vi "ClassesOverview.vi"() -> (0 "error out":errorcluster)   [LabVIEW 2016]
uses:
  <resource>/Framework/Providers/Open_GDS/ClassProviders/Common/LvClass_class/GDSLvCLass_ClassSettingsType.ctl
  <resource>/Framework/Providers/Open_GDS/ClassProviders/Common/LvClass_class/GDSLvClass_PlugIn.ctl
  <resource>/Framework/Providers/Open_GDS/ClassProviders/Common/LvClass_class/GDSLvClass_PlugInTypes.ctl
  <resource>/Framework/Providers/Open_GDS/ClassProviders/Provider_BaseClassInterface/ClassWriter_class/ClassWriter.lvclass
  <vilib>/Utility/miscctls.llb/LVPositionTypeDef.ctl
  <vilib>/Utility/error.llb/DialogType.ctl
panel:
  in  "OnlyClassesThatNeedsToBeUpdated":bool=TRUE
  out "Slide":u8(slide) scale=0.0..100.0
  in  "Done":bool
  in  "UpdateSelected":bool
  in  "Classes":i32[](listbox)
  in  "Cancel":bool
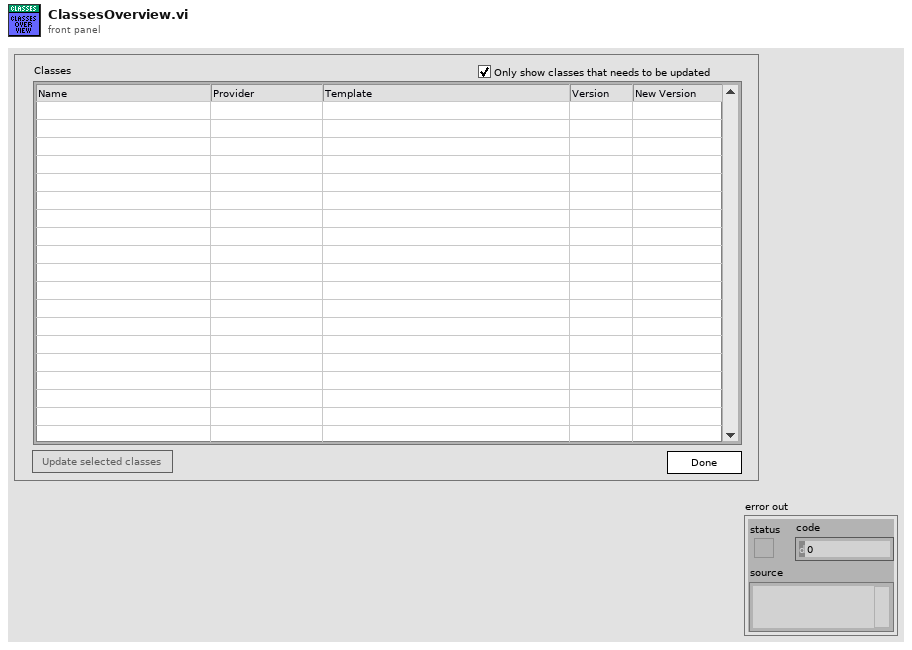
[diagram p1: front panel]
types:
  T1 = typedef "GDSLvCLass_ClassSettingsType.ctl" = cluster{"ClassProviderName":string, "ClassTemplateUsed":string, "ClassTemplateVersion":string, "ClassDescription":string, "PlugIns":T2[], "ConnectorPanePattern":string}
  T2 = typedef "GDSLvClass_PlugIn.ctl" = cluster{"Type":T3, "ID":string, "Version":string, "Path":path, "Name":string, "Data":variant}
  T3 = typedef "GDSLvClass_PlugInTypes.ctl" = enum16{"DesignPattern", "MethodTypes"}
  T4 = cluster{"ClassInfo":T1[], "Classes":refnum<vi>[], "NewVersions":string[], "ClassWriters":refnum<class "ClassWriter.lvclass">[]}
  T5 = typedef "LVPositionTypeDef.ctl" = cluster{"Left":i32, "Top":i32}
  T6 = cluster{"Major":u16, "Minor":u16, "Fix":u16, "Build":u16}
  T7 = typedef "DialogType.ctl" = u16
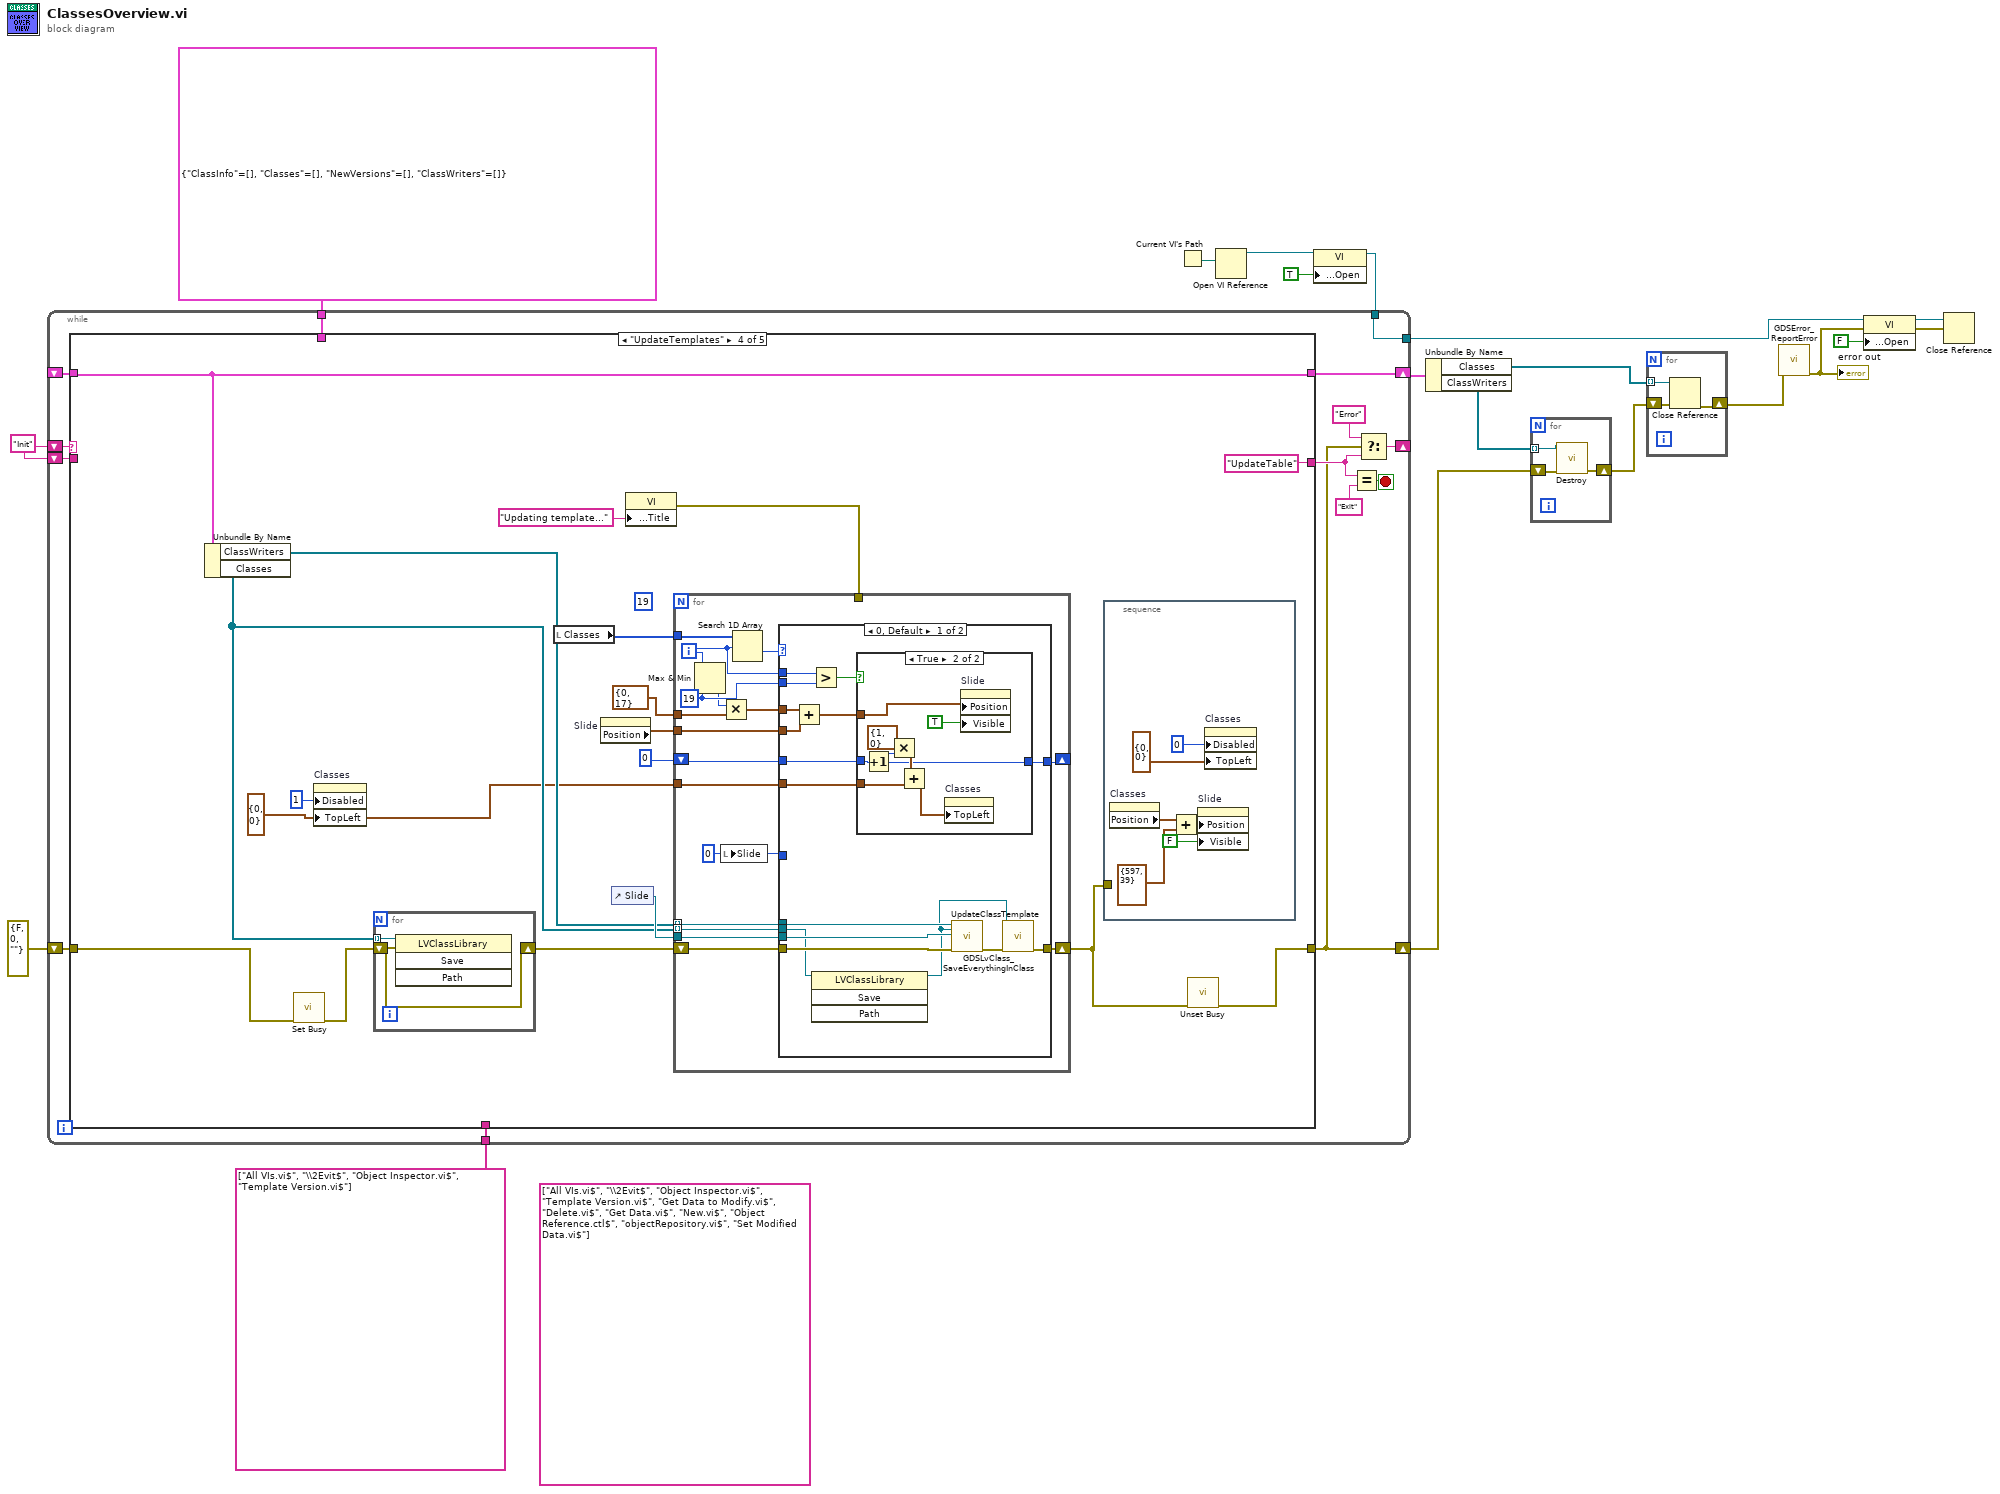
[diagram p0: block diagram]
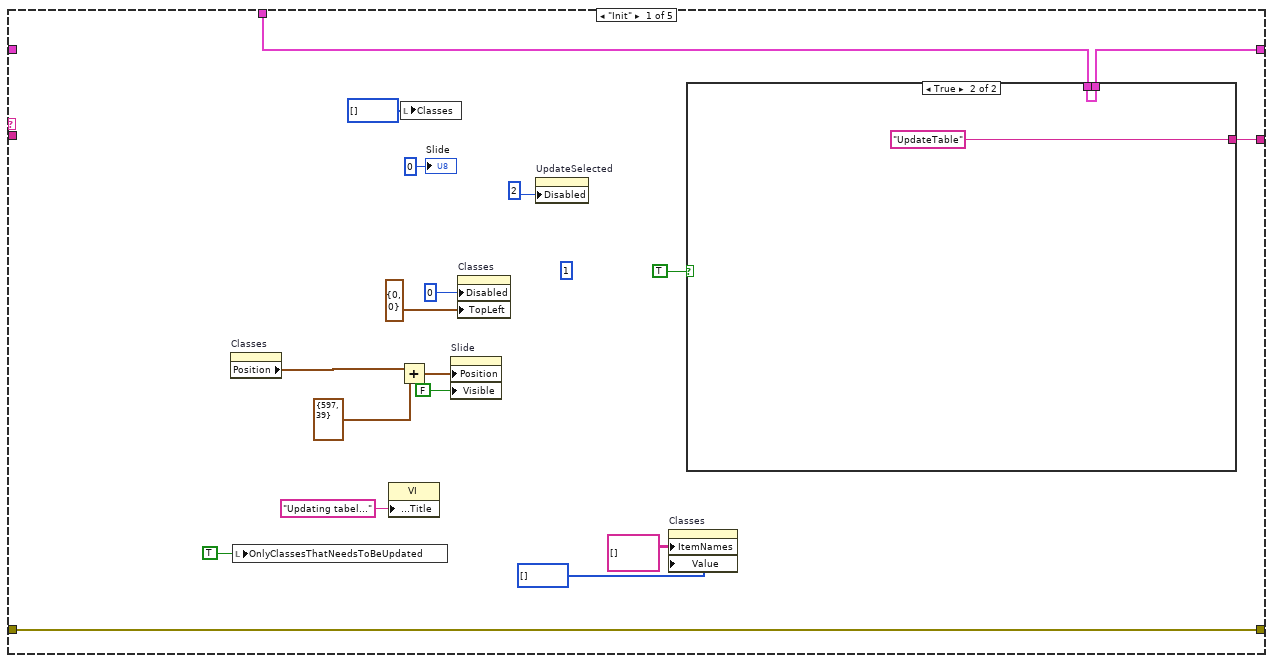
[diagram p2: hidden frame]
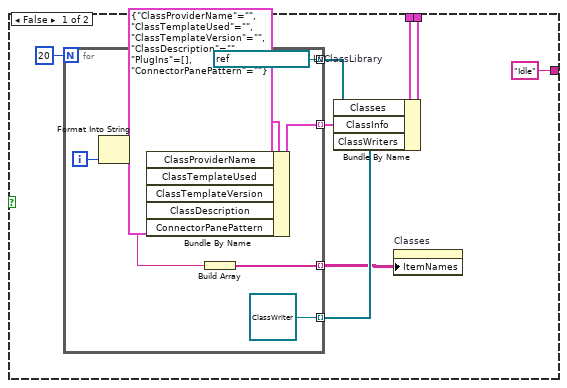
[diagram p3: hidden frame]
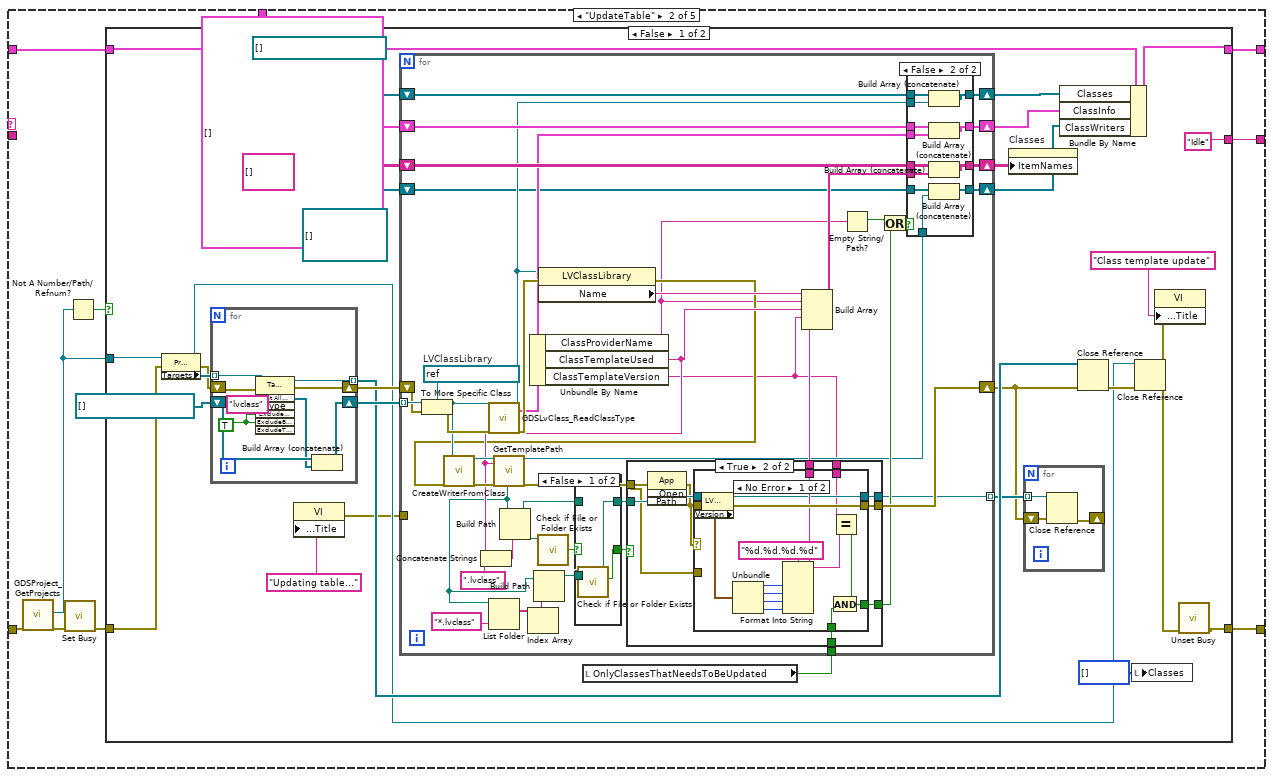
[diagram p4: hidden frame]
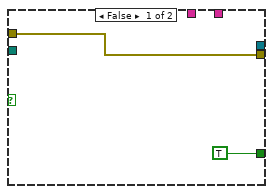
[diagram p6: hidden frame]
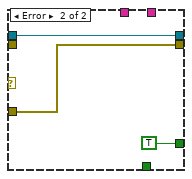
[diagram p7: hidden frame]
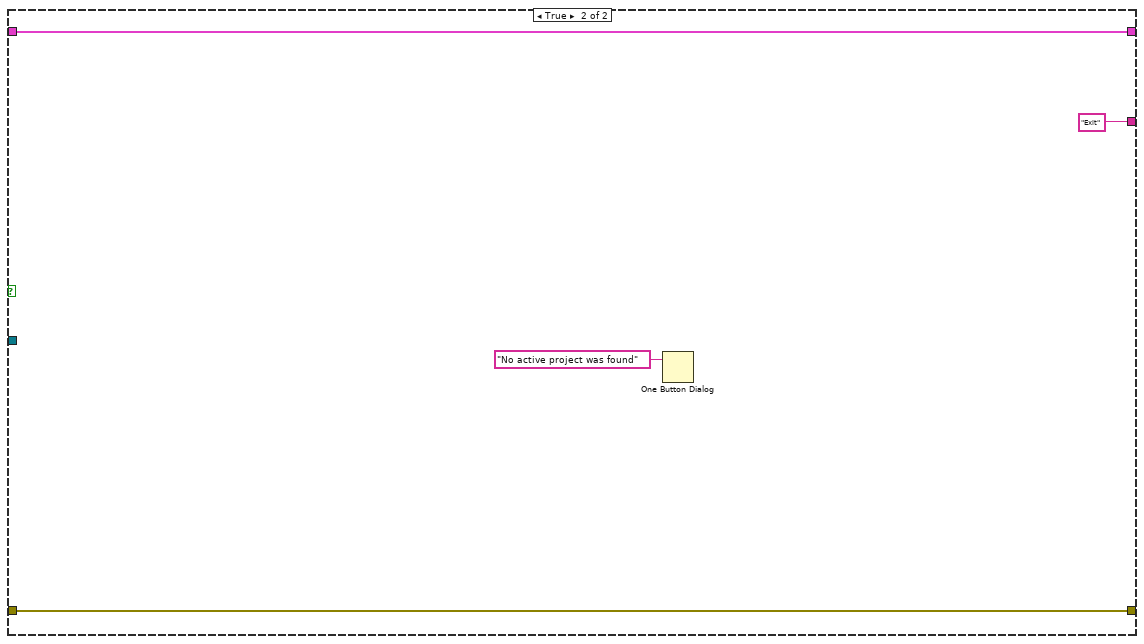
[diagram p9: hidden frame]
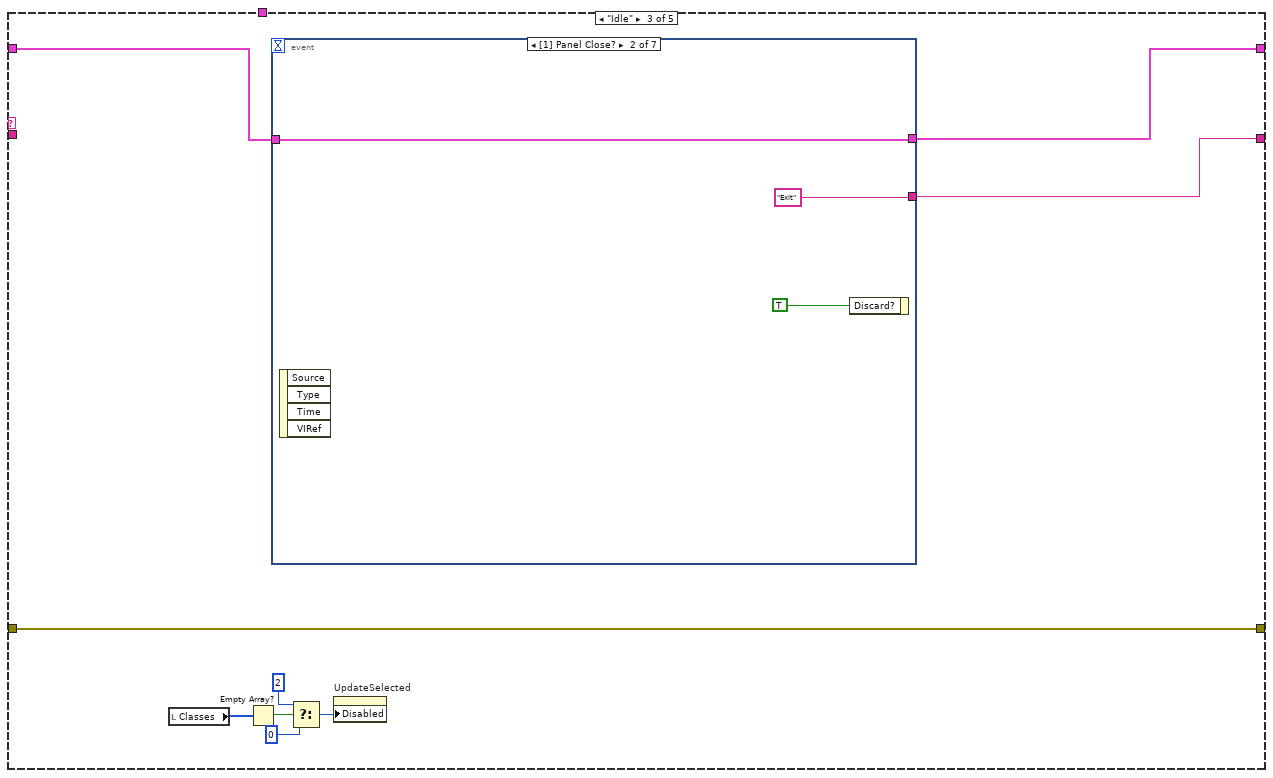
[diagram p10: hidden frame]
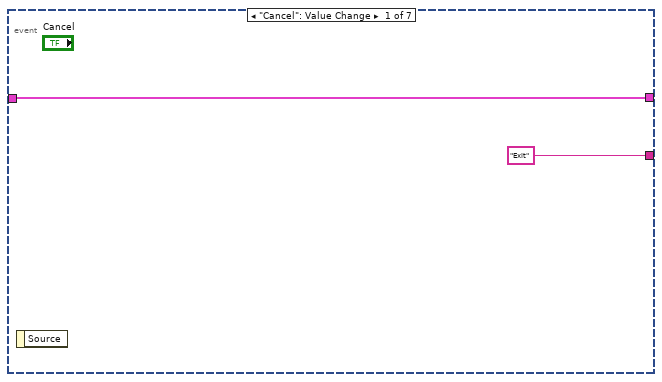
[diagram p11: hidden frame]
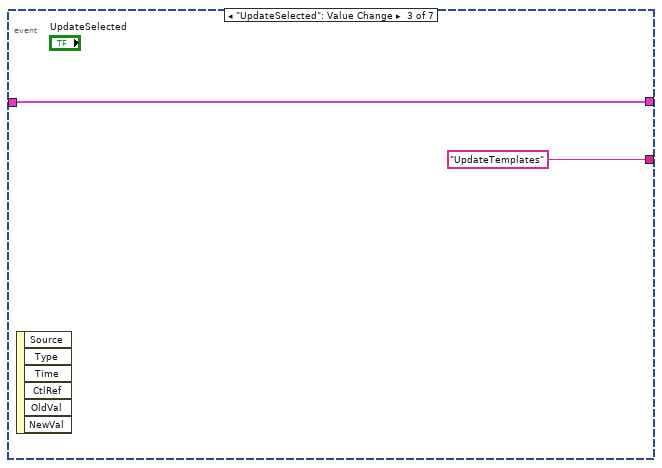
[diagram p12: hidden frame]
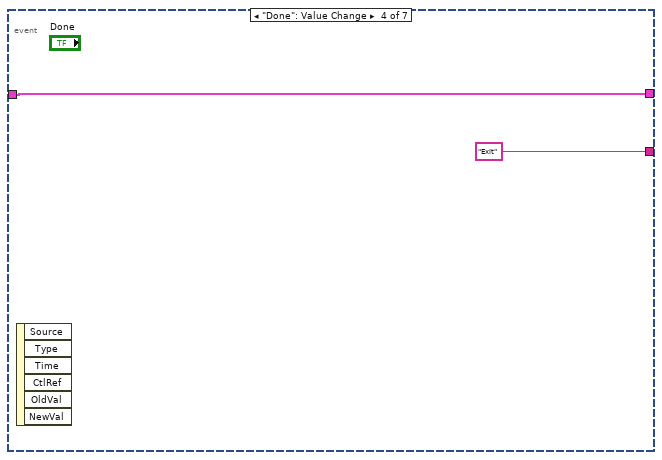
[diagram p13: hidden frame]
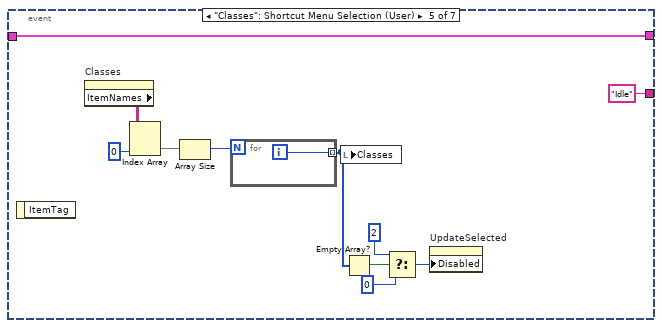
[diagram p14: hidden frame]
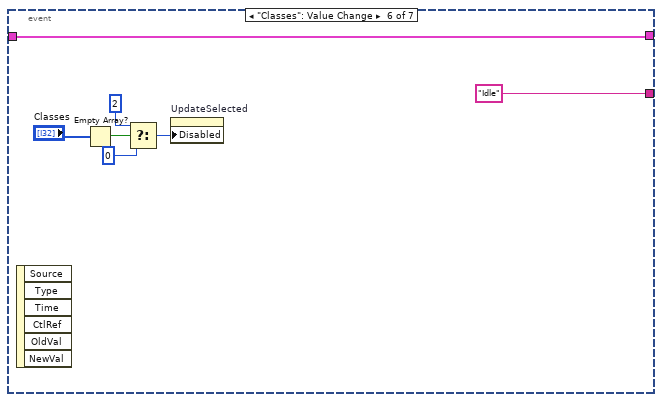
[diagram p15: hidden frame]
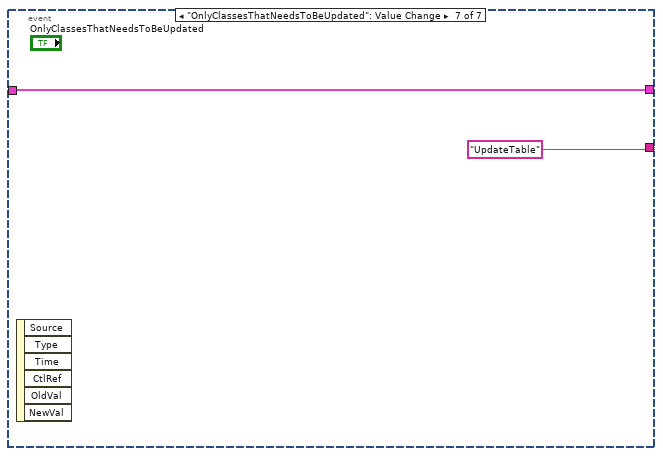
[diagram p16: hidden frame]
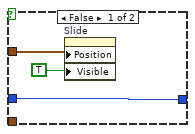
[diagram p17: hidden frame]
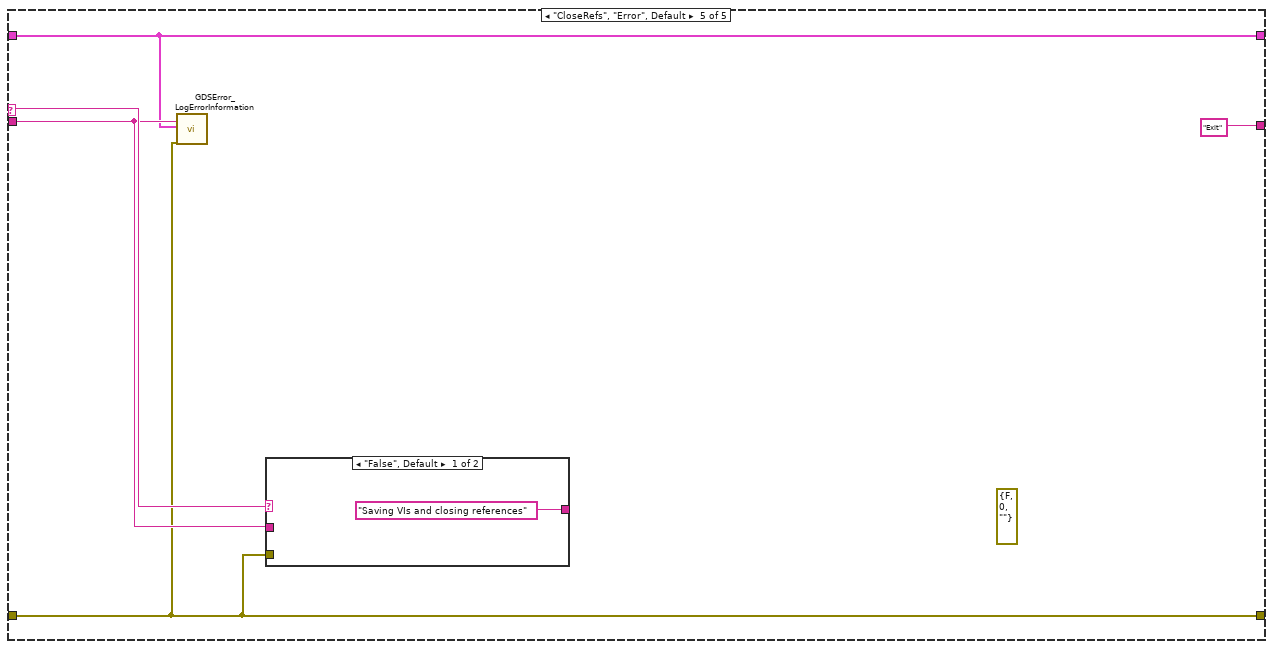
[diagram p19: hidden frame]
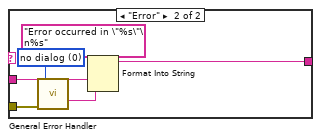
[diagram p20: hidden frame]
diagram:
  (unwired) string[] ["All VIs.vi$", "\\2Evit$", "Object Inspector.vi$", "Template Version.vi$", "Get Data to Modify.vi$", "Delete.vi$", "Get Data.vi$", "New.vi$", "Object Reference.ctl$", "objectRepository.vi$", "Set Modified Data.vi$"] ("file names")
  w17 = "Init"
  n1 = Current VI's Path() -> (path=w16:path)
  n2 = Open VI Reference(vi path=w16) -> (vi reference=w15:refnum<vi>)  [unwired: 5 in, 1 out]
  n3 = property class="VI"(reference=w15, "Front Panel.Open"=TRUE ("Front Panel Window:Open")) -> (reference out=w14:refnum<vi>)  [unwired: 1 in, 1 out]
  n4 = while {
    shift-right: [w27] -> w3
    shift-left: errorcluster {"status"=FALSE, "code"=0, "source"=""} ("error IO") -> [w33]
    shift-right: [w32] -> _
    shift-left: w17 -> [w21]
    shift-right: [w26] -> w6
    shift-left: _ -> [w25]
    tunnel: T4 {"ClassInfo"=[], "Classes"=[], "NewVersions"=[], "ClassWriters"=[]} -> [w24]
    tunnel: string[] ["All VIs.vi$", "\\2Evit$", "Object Inspector.vi$", "Template Version.vi$"] ("file names") -> [w23]
    shift-left: w17 -> [w22]
    tunnel: w14 -> [w20]
    tunnel: [w20] -> w9
    stop <- w31 stop-if-true
    n5 = case shown="\"UpdateTemplates\"" w21 {
      selector: w21 -> [_ _ _ _ w333]
      tunnel: w33 -> [w51 w77 w224 w263 w330]
      tunnel: [w51 w74 w224 w265 w330] -> w27
      tunnel: [w47 w75 w225 "UpdateTable" "Exit"] -> w28
      tunnel: [w38 w73 w226 w275 w331] -> w26
      tunnel: w25 -> [_ w72 w227 w275 w331]
      tunnel: w24 -> [w39 _ _ _ _]
      tunnel: w23 -> [_ _ _ _ _]
      tunnel: w22 -> [_ _ _ _ w332]
      frame "Init" {
        (unwired) u8 1 ("Disabled")
        n6 = property on="Classes" class="MCListbox (strict)"() -> ("Position"=w42:T5)  [unwired: 2 in, 2 out]
        n7 = local write "OnlyClassesThatNeedsToBeUpdated"(TRUE ("OnlyClassesThatNeedsToBeUpdated")) -> ()
        n8 = property class="VI"("Front Panel.Title"="Updating tabel..." ("Front Panel Window:Title")) -> ()  [unwired: 2 in, 2 out]
        n9 = Add(x=w42, y=T5 {"Left"=597, "Top"=39} ("x-y")) -> (x+y=w50:T5)
        n10 = local write "Classes"(i32[] [] ("Classes")) -> ()
        n11 = property on="Slide" class="Slide (strict)"("Position"=w50, "Visible"=FALSE) -> ()  [unwired: 2 in, 2 out]
        n12 = property on="Classes" class="MCListbox (strict)"("Disabled"=u8 0, "TopLeft"=cluster{"Row":u32, "Column":u32} {"Row"=0, "Column"=0} ("Top Left Visible Cell")) -> ()  [unwired: 2 in, 2 out]
        n13 = property on="UpdateSelected" class="Bool"("Disabled"=u8 2) -> ()  [unwired: 2 in, 2 out]
        n14 = property on="Classes" class="MCListbox (strict)"("ItemNames"=string[][] [] ("Item Names"), "Value"=i32[] [] ("Classes")) -> ()  [unwired: 2 in, 2 out]
        n15 = case shown="True" TRUE {
          tunnel: ["Idle" "UpdateTable"] -> w47
          tunnel: w39 -> [w58 w67]
          tunnel: [w57 w67] -> w38
          frame False {
            n16 = for {
              N: 20 -> [_]
              tunnel: [w66] -> w55 mode=indexing
              tunnel: [refnum<class "ClassWriter.lvclass"> refnum ("ClassWriterOut")] -> w54 mode=indexing
              tunnel: [w63] -> w53 mode=indexing
              tunnel: [w60] -> w52 mode=indexing
              i -> [w62]
              w66 = refnum<vi> refnum  # LVClassLibrary
              n17 = Format Into String(w62) -> (resulting string=w61:string)  [unwired: 3 in, 1 out]
              n18 = Bundle By Name(cluster=T1 {"ClassProviderName"="", "ClassTemplateUsed"="", "ClassTemplateVersion"="", "ClassDescription"="", "PlugIns"=[], "ConnectorPanePattern"=""} ("input cluster"), "ClassProviderName"=w61, "ClassTemplateUsed"=w61, "ClassTemplateVersion"=w61, "ClassDescription"=w61, "ConnectorPanePattern"=w61) -> (w63:T1)
              n19 = Build Array(w61) -> (w60:string[])
            }
            n20 = Bundle By Name(cluster=w58, "Classes"=w55, "ClassInfo"=w53, "ClassWriters"=w54) -> (w57:T4)
            n21 = property on="Classes" class="MCListbox (strict)"("ItemNames"=w52) -> ()  [unwired: 2 in, 2 out]
          }
          frame True {
          }
        }
        "Slide" <- u8 0 ("Slide")
      }
      frame "UpdateTable" {
        n22 = call <resource>:"GDSProject_GetProjects.vi"("error in (no error)"=w77) -> ("Project Refnum"=w71:refnum<vi>, "error out"=w70:errorcluster)  [unwired: 16 in, 1 out]
        n23 = call <vilib>:"Set Busy.vi"("error in (no error)"=w70) -> ("error out"=w69:errorcluster)  [unwired: 9 in, 1 out]
        n24 = Not A Number/Path/Refnum?(number/path/refnum=w71) -> (NaN/Path/Refnum?=w76:bool)
        n25 = case shown="False" w76 {
          tunnel: w69 -> [w106 w217]
          tunnel: ["Idle" "Exit"] -> w75
          tunnel: [w80 w217] -> w74
          tunnel: [w98 w215] -> w73
          tunnel: w72 -> [w102 w215]
          tunnel: w71 -> [w107 _]
          frame False {
            n26 = property class="Project"(reference=w107, error in=w106) -> (reference out=w99:refnum<vi>, error out=w78:errorcluster, "Targets"=w105:refnum<vi>[])
            n27 = for {
              tunnel: w105 -> [w116] mode=indexing
              tunnel: [w111] -> w101 mode=indexing
              shift-right: [w108] -> w104
              shift-left: refnum<vi>[] [] -> [w110]
              shift-right: [w112] -> w103
              shift-left: w78 -> [w114]
              w113 = TRUE ("ExcludeDependencies")
              n28 = invoke class="TargetItem" method="Get All Descendents"(reference=w116, error in=w114, "Type"="lvclass", "Exclude Dependencies"=w113, "ExcludeBuilds"=w113) -> (reference out=w111:refnum<vi>, error out=w112:errorcluster, "All Descendents"=w109:refnum<vi>[])  [unwired: 2 in, 4 out]
              n29 = Build Array (concatenate)(w110, w109) -> (w108:refnum<vi>[])
            }
            n30 = property class="VI"("Front Panel.Title"="Updating table..." ("Front Panel Window:Title")) -> (error out=w82:errorcluster)  [unwired: 2 in, 1 out]
            n31 = local read "OnlyClassesThatNeedsToBeUpdated"() -> (w86:bool)
            n32 = for {
              tunnel: w104 -> [w163] mode=indexing
              shift-right: [w140] -> w91
              shift-left: w103 -> [w161]
              shift-right: [w156] -> w97
              shift-left: string[][] [] -> [w157]
              shift-right: [w154] -> w89
              shift-left: T1[] [] ("ClassInfo") -> [w153]
              shift-right: [w151] -> w93
              shift-left: refnum<vi>[] [] ("Classes") -> [w152]
              tunnel: [w134] -> w92 mode=indexing
              shift-right: [w132] -> w87
              shift-left: refnum<class "ClassWriter.lvclass">[] [] ("ClassWriters") -> [w133]
              tunnel: w86 -> [w129]
              tunnel: w82 -> [_]
              w162 = refnum<vi> refnum  # LVClassLibrary
              n33 = To More Specific Class(target class=w162, reference=w163, error in=w161) -> (specific class reference=w143:refnum<vi>, error out=w160:errorcluster)
              n34 = call <resource>:"GDSLvClass_ReadClassType.vi"("Class Refnum In"=w143, "error in (no error)"=w160) -> ("Class Refnum Out"=w149:refnum<vi>, "ClassSettings"=w150:T1, "error out"=w158:errorcluster)  [unwired: 15 in]
              n35 = Unbundle By Name(w150) -> ("ClassProviderName"=w138:string, "ClassTemplateUsed"=w142:string, "ClassTemplateVersion"=w130:string)
              n36 = Concatenate Strings(w142, ".lvclass" ("string")) -> (w148:string)
              n37 = property class="LVClassLibrary"(reference=w149, error in=w158) -> (error out=w141:errorcluster, "Name"=w159:string)  [unwired: 1 out]
              n38 = call <resource>:"CreateWriterFromClass.vi"("ClassPath/LvClassRef"=w143, "error in"=w141) -> ("ClassWriter"=w145:refnum<class "ClassWriter.lvclass">, "error out"=w144:errorcluster)  [unwired: 15 in, 1 out]
              n39 = call-dynamic "GetTemplatePath.vi"("ClassWriterIn"=w145, "ClassTemplateSubDirectory"=w142, "error in (no error)"=w144) -> ("ClassWriterOut"=w131:refnum<class "ClassWriter.lvclass">, "FolderPathOut"=w121:path, "error out"=w146:errorcluster)  [unwired: 12 in, 2 out]
              n40 = List Folder(path=w121, pattern="*.lvclass" ("string")) -> (filenames=w123:string[])  [unwired: 2 in, 3 out]
              n41 = Build Path(base path=w121, name or relative path=w148) -> (appended path=w126:path)
              n42 = Index Array(array=w123) -> (element=w122:string)  [unwired: 1 in]
              n43 = Build Path(base path=w121, name or relative path=w122) -> (appended path=w120:path)
              n44 = call <vilib>:"Check if File or Folder Exists.vi"("path"=w126) -> ("file or folder exists?"=w127:bool)  [unwired: 8 in, 2 out]
              n45 = case shown="False" w127 {
                selector: w127 -> [_ w168]
                tunnel: w126 -> [_ w167]
                tunnel: [w165 w168] -> w125
                tunnel: [w164 w167] -> w124
                tunnel: w120 -> [w166 _]
                frame False {
                  n46 = call <vilib>:"Check if File or Folder Exists.vi"("path"=w166) -> ("file or folder exists?"=w165:bool, "dup path"=w164:path)  [unwired: 8 in, 1 out]
                }
                frame True {
                }
              }
              n47 = case shown="True" w125 {
                tunnel: w146 -> [w170 w171]
                tunnel: [w170 w179] -> w140
                tunnel: [_ w178] -> w139
                tunnel: [TRUE w177] -> w135
                tunnel: [_ w176] -> w134
                tunnel: w130 -> [_ w175]
                tunnel: w124 -> [_ w174]
                tunnel: w129 -> [_ w173]
                frame False {
                }
                frame True {
                  n48 = invoke class="App" method="LVClass.Open"(error in=w171, "Path"=w174) -> (error out=w172:errorcluster, "LVClass.Open"=w180:refnum<vi>)  [unwired: 2 in, 2 out]
                  n49 = case shown="No Error" w172 {
                    tunnel: w180 -> [w195 w198]
                    tunnel: w172 -> [w188 _]
                    tunnel: [w187 w197] -> w179
                    tunnel: [w186 _] -> w178
                    tunnel: [w184 TRUE] -> w177
                    tunnel: [w183 w198] -> w176
                    tunnel: w175 -> [w182 _]
                    tunnel: w173 -> [w181 _]
                    tunnel: w171 -> [_ w197]
                    frame No Error {
                      n50 = property class="LVClassLibrary"(reference=w195, error in=w188) -> (reference out=w183:refnum<vi>, error out=w187:errorcluster, "Version"=w189:T6)
                      n51 = Unbundle(w189) -> ("Major"=w194:u16, "Minor"=w193:u16, "Fix"=w192:u16, "Build"=w191:u16)
                      n52 = Format Into String(format string="%d.%d.%d.%d", w194, w193, w192, w191) -> (resulting string=w186:string)  [unwired: 2 in, 1 out]
                      n53 = Equal?(x=w182, y=w186) -> (x = y?=w185:bool)
                      n54 = And(x=w185, y=w181) -> (x .and. y?=w184:bool)
                    }
                    frame Error {
                    }
                  }
                }
              }
              n55 = Build Array(w159, w138, w142, w130, w139) -> (w155:string[])
              n56 = Empty String/Path?(string/path=w138) -> (empty?=w137:bool)
              n57 = Or(x=w137, y=w135) -> (x .or. y?=w136:bool)
              n58 = case shown="False" w136 {
                tunnel: w157 -> [w202 w214]
                tunnel: [w202 w213] -> w156
                tunnel: w155 -> [_ w212]
                tunnel: w153 -> [w200 w210]
                tunnel: [w200 w211] -> w154
                tunnel: w152 -> [w201 w209]
                tunnel: [w201 w208] -> w151
                tunnel: w149 -> [_ w207]
                tunnel: w150 -> [_ w206]
                tunnel: w133 -> [w199 w205]
                tunnel: [w199 w204] -> w132
                tunnel: w131 -> [_ w203]
                frame True {
                }
                frame False {
                  n59 = Build Array (concatenate)(w209, w207) -> (w208:refnum<vi>[])
                  n60 = Build Array (concatenate)(w210, w206) -> (w211:T1[])
                  n61 = Build Array (concatenate)(w214, w212) -> (w213:string[][])
                  n62 = Build Array (concatenate)(w205, w203) -> (w204:refnum<class "ClassWriter.lvclass">[])
                }
              }
            }
            n63 = property on="Classes" class="MCListbox (strict)"("ItemNames"=w97) -> ()  [unwired: 2 in, 2 out]
            n64 = for {
              tunnel: w92 -> [w118] mode=indexing
              shift-right: [w117] -> _
              shift-left: w91 -> [w119]
              n65 = Close Reference(reference=w118, error in (no error)=w119) -> (error out=w117:errorcluster)
            }
            n66 = Bundle By Name(cluster=w102, "Classes"=w93, "ClassInfo"=w89, "ClassWriters"=w87) -> (w98:T4)
            n67 = Close Reference(reference=w101, error in (no error)=w91) -> (error out=w100:errorcluster)
            n68 = local write "Classes"(i32[] [] ("Classes")) -> ()
            n69 = Close Reference(reference=w99, error in (no error)=w100) -> (error out=w81:errorcluster)
            n70 = property class="VI"(error in=w81, "Front Panel.Title"="Class template update" ("Front Panel Window:Title")) -> ()  [unwired: 1 in, 2 out]
            n71 = call <vilib>:"Unset Busy.vi"("error in (no error)"=w81) -> ("error out"=w80:errorcluster)  [unwired: 10 in]
          }
          frame True {
            n72 = One Button Dialog(message="No active project was found") -> ()  [unwired: 1 in, 1 out]
          }
        }
      }
      frame "Idle" {
        n73 = local read "Classes"() -> (w219:i32[])
        n74 = Empty Array?(array=w219) -> (empty?=w220:bool)
        n75 = event shown="[1] Panel Close?" {
          selector: _ -> [_ _ _ _ _ _ _]
          dyn-events: _ -> [_ _ _ _ _ _ _]
          timeout: _ -> [_ _ _ _ _ _ _]
          tunnel: w227 -> [w228 w230 w234 w236 w243 w255 w256]
          tunnel: [w228 w230 w234 w236 w243 w255 w256] -> w226
          tunnel: ["Exit" "Exit" "UpdateTemplates" "Exit" "Idle" "Idle" "UpdateTable"] -> w225
          event "Cancel": Value Change {
            n76 = event-data() -> ()  [unwired: 1 in, 1 out]
          }
          event Panel Close? {
            n77 = event-data() -> ()  [unwired: 1 in, 4 out]
            n78 = event-data("Discard?"=TRUE ("Front Panel Window:Open")) -> ()  [unwired: 1 in, 1 out]
          }
          event "UpdateSelected": Value Change {
            n79 = event-data() -> ()  [unwired: 1 in, 6 out]
          }
          event "Done": Value Change {
            n80 = event-data() -> ()  [unwired: 1 in, 6 out]
          }
          event "Classes": Shortcut Menu Selection (User) {
            n81 = event-data() -> ()  [unwired: 1 in, 1 out]
            n82 = property on="Classes" class="MCListbox (strict)"() -> ("ItemNames"=w247:string[][])  [unwired: 2 in, 2 out]
            n83 = Index Array(array=w247, index (col)=0 ("disabled index (col)")) -> (element=w245:string[])  [unwired: 1 in]
            n84 = Array Size(array=w245) -> (size(s)=w244:i32)
            n85 = for {
              N: w244 -> [_]
              tunnel: [w248] -> w238 mode=indexing
              i -> [w248]
            }
            n86 = local write "Classes"(w238) -> ()
            n87 = Empty Array?(array=w238) -> (empty?=w242:bool)
            n88 = Select(t=u8 2 ("Disabled"), s=w242, f=u8 0) -> (s? t:f=w240:u8)
            n89 = property on="UpdateSelected" class="Bool"("Disabled"=w240) -> ()  [unwired: 2 in, 2 out]
          }
          event "Classes": Value Change {
            n90 = event-data() -> ()  [unwired: 1 in, 6 out]
            n91 = Empty Array?(array="Classes") -> (empty?=w253:bool)
            n92 = Select(t=u8 2 ("Disabled"), s=w253, f=u8 0) -> (s? t:f=w251:u8)
            n93 = property on="UpdateSelected" class="Bool"("Disabled"=w251) -> ()  [unwired: 2 in, 2 out]
          }
          event "OnlyClassesThatNeedsToBeUpdated": Value Change {
            n94 = event-data() -> ()  [unwired: 1 in, 6 out]
          }
        }
        n95 = Select(t=u8 2 ("Disabled"), s=w220, f=u8 0) -> (s? t:f=w222:u8)
        n96 = property on="UpdateSelected" class="Bool"("Disabled"=w222) -> ()  [unwired: 2 in, 2 out]
      }
      frame "UpdateTemplates" {
        w258 = cluster{"Row":u32, "Column":u32} {"Row"=0, "Column"=0} ("Top Left Visible Cell")
        (unwired) 19
        n97 = Unbundle By Name(w275) -> ("ClassWriters"=w268:refnum<class "ClassWriter.lvclass">[], "Classes"=w264:refnum<vi>[])
        n98 = call <vilib>:"Set Busy.vi"("error in (no error)"=w263) -> ("error out"=w261:errorcluster)  [unwired: 9 in, 1 out]
        n99 = property on="Classes" class="MCListbox (strict)"("Disabled"=u8 1, "TopLeft"=w258) -> ()  [unwired: 2 in, 2 out]
        n100 = for {
          tunnel: w264 -> [w277] mode=indexing
          shift-right: [w276] -> w262
          shift-left: w261 -> [w276]
          n101 = invoke class="LVClassLibrary" method="Save"(reference=w277, error in=w276) -> ()  [unwired: 2 in, 4 out]
        }
        n102 = local read "Classes"() -> (w274:i32[])
        n103 = property on="Slide" class="Slide (strict)"() -> ("Position"=w271:T5)  [unwired: 2 in, 2 out]
        n104 = control-ref of="Slide"() -> (w273:refnum<vi>)
        n105 = property class="VI"("Front Panel.Title"="Updating template..." ("Front Panel Window:Title")) -> (error out=w259:errorcluster)  [unwired: 2 in, 1 out]
        n106 = for {
          shift-right: [w299] -> w266
          shift-left: w262 -> [w300]
          tunnel: w268 -> [w298] mode=indexing
          tunnel: w264 -> [w297] mode=indexing
          tunnel: w274 -> [w296]
          tunnel: w273 -> [w294]
          tunnel: T5 {"Left"=0, "Top"=17} ("y") -> [w293]
          tunnel: w271 -> [w291]
          tunnel: w258 -> [w290]
          shift-right: [w288] -> _
          shift-left: u32 0 ("Left") -> [w289]
          tunnel: w259 -> [_]
          i -> [w287]
          w284 = u8 0 ("Left")
          w286 = 19 ("y")
          n107 = Max & Min(x=w287, y=w286) -> (min(x,y)=w285:i32)  [unwired: 1 out]
          n108 = Multiply(x=w285, y=w293) -> (x*y=w292:T5)
          n109 = local write "Slide"(w284) -> ()
          n110 = Search 1D Array(1D array=w296, element=w287) -> (index of element=w295:i32)  [unwired: 1 in]
          n111 = case shown="0, Default" w295 {
            tunnel: w300 -> [w315 w329]
            tunnel: [w314 w329] -> w299
            tunnel: w298 -> [w316 _]
            tunnel: w297 -> [w302 _]
            tunnel: w294 -> [w313 _]
            tunnel: w292 -> [w312 _]
            tunnel: w291 -> [w311 _]
            tunnel: w287 -> [w309 _]
            tunnel: w290 -> [w307 _]
            tunnel: w289 -> [w306 w328]
            tunnel: [w305 w328] -> w288
            tunnel: w286 -> [w304 _]
            tunnel: w284 -> [_ _]
            frame 0, Default {
              n112 = Add(x=w312, y=w311) -> (x+y=w310:T5)
              n113 = Greater?(x=w309, y=w304) -> (0:w308:bool)
              n114 = invoke class="LVClassLibrary" method="Save"(reference=w302) -> (reference out=w301:refnum<vi>)  [unwired: 3 in, 3 out]
              n115 = case shown="True" w308 {
                tunnel: w310 -> [w319 w320]
                tunnel: w307 -> [_ w327]
                tunnel: w306 -> [w317 w323]
                tunnel: [w317 w322] -> w305
                frame False {
                  n116 = property on="Slide" class="Slide (strict)"("Position"=w319, "Visible"=TRUE) -> ()  [unwired: 2 in, 2 out]
                }
                frame True {
                  n117 = Increment(x=w323) -> (x+1=w322:u32)
                  n118 = Multiply(x=cluster{"Left":u32, "Top":u32} {"Left"=1, "Top"=0} ("y"), y=w322) -> (x*y=w325:cluster{"Left":u32, "Top":u32})
                  n119 = Add(x=w325, y=w327) -> (x+y=w324:cluster{u32, u32})
                  n120 = property on="Classes" class="MCListbox (strict)"("TopLeft"=w324) -> ()  [unwired: 2 in, 2 out]
                  n121 = property on="Slide" class="Slide (strict)"("Position"=w320, "Visible"=TRUE) -> ()  [unwired: 2 in, 2 out]
                }
              }
              n122 = call-dynamic "UpdateClassTemplate.vi"("ClassWriterIn"=w316, "LVClassLibraryRef"=w301, "ProgressBar"=w313, "error in (no error)"=w315) -> ("error out"=w303:errorcluster)  [unwired: 14 in, 1 out]
              n123 = call <resource>:"GDSLvClass_SaveEverythingInClass.vi"("ClassRefIn"=w301, "error in"=w303) -> ("error out"=w314:errorcluster)  [unwired: 16 in, 1 out]
            }
            frame -1 {
            }
          }
        }
        n124 = stacked-sequence {
          tunnel: w266 -> [_]
          frame #0 {
            n125 = property on="Classes" class="MCListbox (strict)"() -> ("Position"=w283:T5)  [unwired: 2 in, 2 out]
            n126 = Add(x=w283, y=T5 {"Left"=597, "Top"=39} ("x-y")) -> (x+y=w282:T5)
            n127 = property on="Slide" class="Slide (strict)"("Position"=w282, "Visible"=FALSE) -> ()  [unwired: 2 in, 2 out]
            n128 = property on="Classes" class="MCListbox (strict)"("Disabled"=u8 0, "TopLeft"=cluster{"Row":u32, "Column":u32} {"Row"=0, "Column"=0} ("Top Left Visible Cell")) -> ()  [unwired: 2 in, 2 out]
          }
        }
        n129 = call <vilib>:"Unset Busy.vi"("error in (no error)"=w266) -> ("error out"=w265:errorcluster)  [unwired: 10 in]
      }
      frame "CloseRefs", "Error", Default {
        (unwired) errorcluster {"status"=FALSE, "code"=0, "source"=""} ("error IO")
        n130 = call <resource>:"GDSError_LogErrorInformation.vi"("State"=w332, "LocalVariableData"=w331, "error in (no error)"=w330) -> ()  [unwired: 16 in, 1 out]
        n131 = case shown="\"False\", Default" w333 {
          tunnel: w332 -> [_ w340]
          tunnel: w330 -> [_ w338]
          tunnel: ["Saving VIs and closing references" w336] -> _
          frame "False", Default {
          }
          frame "Error" {
            w339 = T7 0 items=["no dialog", "OK message", "continue or stop message", "OK message + warnings", "continue/stop + warnings"] ("type of dialog (OK msg:1)")
            n132 = call <vilib>:"General Error Handler.vi"("type of dialog (OK msg:1)"=w339, "error in (no error)"=w338) -> ("message"=w337:string)  [unwired: 9 in, 4 out]
            n133 = Format Into String(format string="Error occurred in \"%s\"\n%s", w340, w337) -> (resulting string=w336:string)  [unwired: 2 in, 1 out]
          }
        }
      }
    }
    n134 = Equal?(x=w28, y="Exit") -> (x = y?=w31:bool)
    n135 = Select(t="Error", s=w27, f=w28) -> (s? t:f=w32:string)
  }
  n136 = Unbundle By Name(w6) -> ("Classes"=w5:refnum<vi>[], "ClassWriters"=w1:refnum<class "ClassWriter.lvclass">[])
  n137 = for {
    tunnel: w1 -> [w342] mode=indexing
    shift-right: [w344] -> w2
    shift-left: w3 -> [w343]
    n138 = call-dynamic "Destroy.vi"("ClassWriter.lvclass"=w342, "error in (no error)"=w343) -> ("error out"=w344:errorcluster)  [unwired: 17 in]
  }
  n139 = for {
    tunnel: w5 -> [w347] mode=indexing
    shift-right: [w346] -> w4
    shift-left: w2 -> [w345]
    n140 = Close Reference(reference=w347, error in (no error)=w345) -> (error out=w346:errorcluster)
  }
  n141 = call <resource>:"GDSError_ReportError.vi"("error in (no error)"=w4) -> ("error out"=w11:errorcluster)  [unwired: 18 in]
  "error out" <- w11
  n142 = property class="VI"(reference=w9, error in=w11, "Front Panel.Open"=FALSE ("Front Panel Window:Open")) -> (reference out=w8:refnum<vi>, error out=w10:errorcluster)
  n143 = Close Reference(reference=w8, error in (no error)=w10) -> ()  [unwired: 1 out]
